vi "Run Test Suite.vi"(8 "error in (no error)":errorcluster, 11 "Execution UI In":refnum<class "Execution UI V2.lvclass">) -> (0 "error out":errorcluster, 3 "Execution UI Out":refnum<class "Execution UI V2.lvclass">)   [LabVIEW 2020, in "Execution UI V2.lvclass"]
uses:
  Execution UI V2.lvclass
  Execution UI V2.lvclass/Execution UI V2.ctl
  Application Framework/Process Classes/Process/Process.lvclass/Process.ctl
  Framework/Helper Classes/Result Table/Result Table/Result Table.lvclass/Result Table.ctl
  Application Framework/Process Classes/Process/Protected/Messaging/Enqueue Message.vi
  Framework/Test Runner/Test Runner.lvclass
  C:/Git/astemes-lunit/source/Application Framework/Process Classes/Process/Process.lvclass
  Framework/Helper Classes/Result Table/Result Table/Result Table.lvclass
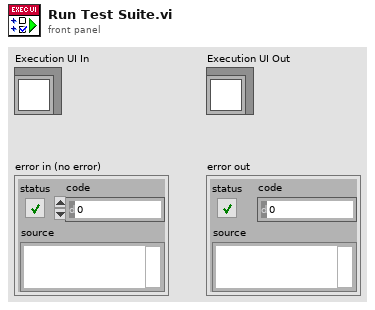
[diagram p1: front panel]
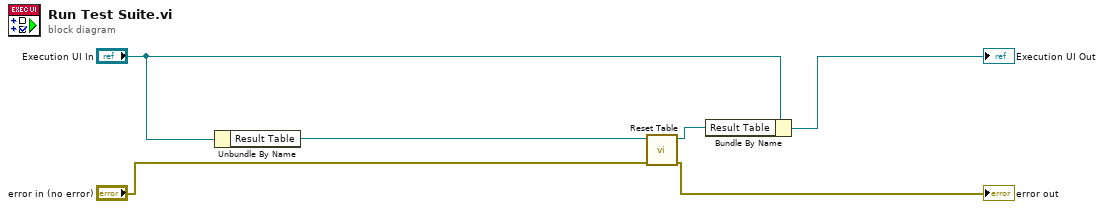
[diagram p0: block diagram]
diagram:
  n1 = Unbundle By Name("Execution UI In") -> ("Result Table"=w3:refnum<class "Result Table.lvclass">)
  n2 = call "Reset Table.vi"("error in (no error)"="error in (no error)", "Result Table.lvclass"=w3) -> ("error out"=→"error out":errorcluster, "Result Table"=w2:refnum<class "Result Table.lvclass">)  [unwired: 8 in]
  n3 = Bundle By Name(cluster="Execution UI In", "Result Table"=w2) -> (→"Execution UI Out":refnum<class "Execution UI V2.lvclass">)
